vi "NI VeriStand - Add Channel Under Section.vi"(8 "Error in":errorcluster, 10 "Channel Ref in":refnum<k24>, 11 "Parent Ref In":refnum<k24>) -> (0 "Error out":errorcluster, 2 "Attached Child Node":bool, 3 "Parent Ref out":refnum<k24>)   [LabVIEW 2025, in "NI_VS RuntimeConfigurationFile ScriptingAPI.lvlib"]
uses:
  NI_VS RuntimeConfigurationFile ScriptingAPI.lvlib
  NationalInstruments.VeriStand.SystemDefinitionAPI
  NationalInstruments.VeriStand.SystemStorage
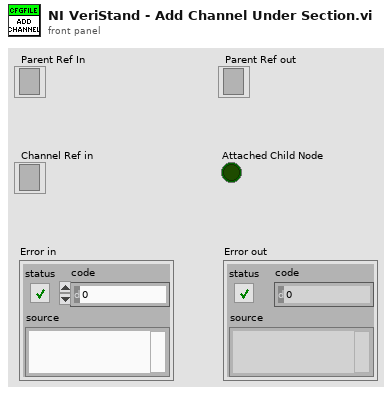
[diagram p1: front panel]
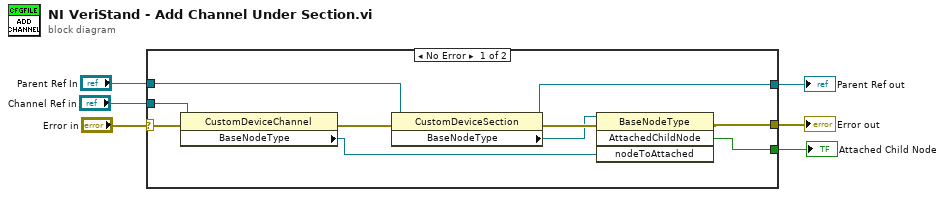
[diagram p0: block diagram]
diagram:
  n1 = case shown="No Error" "Error in" {
    selector: "Error in" -> [w13 w18]
    tunnel: [w14 w18] -> w6
    tunnel: "Parent Ref In" -> [w12 w17]
    tunnel: "Channel Ref in" -> [w11 _]
    tunnel: [w10 w17] -> w2
    tunnel: [w9 _] -> w1
    frame No Error {
      n2 = property class="CustomDeviceChannel"(reference=w11, error in=w13) -> (error out=w16:errorcluster, "BaseNodeType"=w7:refnum<k24>)  [unwired: 1 out]
      n3 = property class="CustomDeviceSection"(reference=w12, error in=w16) -> (reference out=w10:refnum<k24>, error out=w15:errorcluster, "BaseNodeType"=w8:refnum<k24>)
      n4 = invoke class="BaseNodeType" method="AttachedChildNode"(reference=w8, error in=w15, "nodeToAttached"=w7) -> (error out=w14:errorcluster, "AttachedChildNode"=w9:bool)  [unwired: 1 in, 2 out]
    }
    frame Error {
    }
  }
  "Parent Ref out" <- w2
  "Attached Child Node" <- w1
  "Error out" <- w6
